vi "Initialize.vi"(7 "timeout (10000 ms)":i32=10000, 8 "error in (no error)":errorcluster, 10 "API key":string, 11 "server url":string="https://demo.elabftw.net") -> (0 "error out":errorcluster, 3 "eLab out":refnum<class "PL eLabFTW Client.lvclass">)   [LabVIEW 2015, in "PL eLabFTW Client.lvclass"]
doc: "Initializes connection to eLabFTW server using specified settings."
uses:
  PL eLabFTW Client.lvclass
  PL eLabFTW Client.lvclass/PL eLabFTW Client.ctl
  <vilib>/httpClient/LabVIEWHTTPClient.lvlib
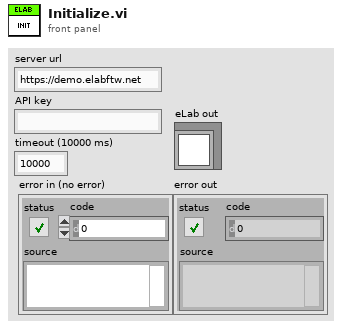
[diagram p1: front panel]
types:
  T1 = typedef "LabVIEWHTTPClient.lvlib/ClientHandle.ctl" = refnum<k1>
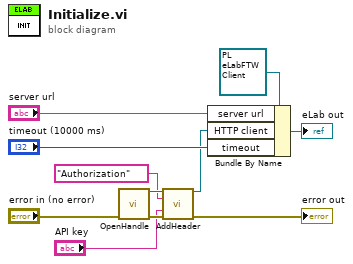
[diagram p0: block diagram]
diagram:
  n1 = call <vilib>:"OpenHandle.vi"("error in (no error)"="error in (no error)") -> ("client handle out"=w7:T1, "error out"=w6:errorcluster)  [unwired: 13 in]
  n2 = call <vilib>:"AddHeader.vi"("client handle"=w7, "header"="Authorization", "value"="API key", "error in (no error)"=w6) -> ("client handle out"=w1:T1, "error out"=→"error out":errorcluster)  [unwired: 10 in]
  n3 = Bundle By Name(cluster=refnum<class "PL eLabFTW Client.lvclass"> refnum, "server url"="server url", "HTTP client"=w1, "timeout"="timeout (10000 ms)") -> (→"eLab out":refnum<class "PL eLabFTW Client.lvclass">)
